vi "ProcAndStates.vi"(0 "spreadsheet string":string) -> (1 "PROCESSES":string[](array[string]), 2 "STATES":string[][](array[string]))   [LabVIEW 2009]
panel:
  out "size(s)":i32[](array[numeric])
  out "Array":string[](array[string])
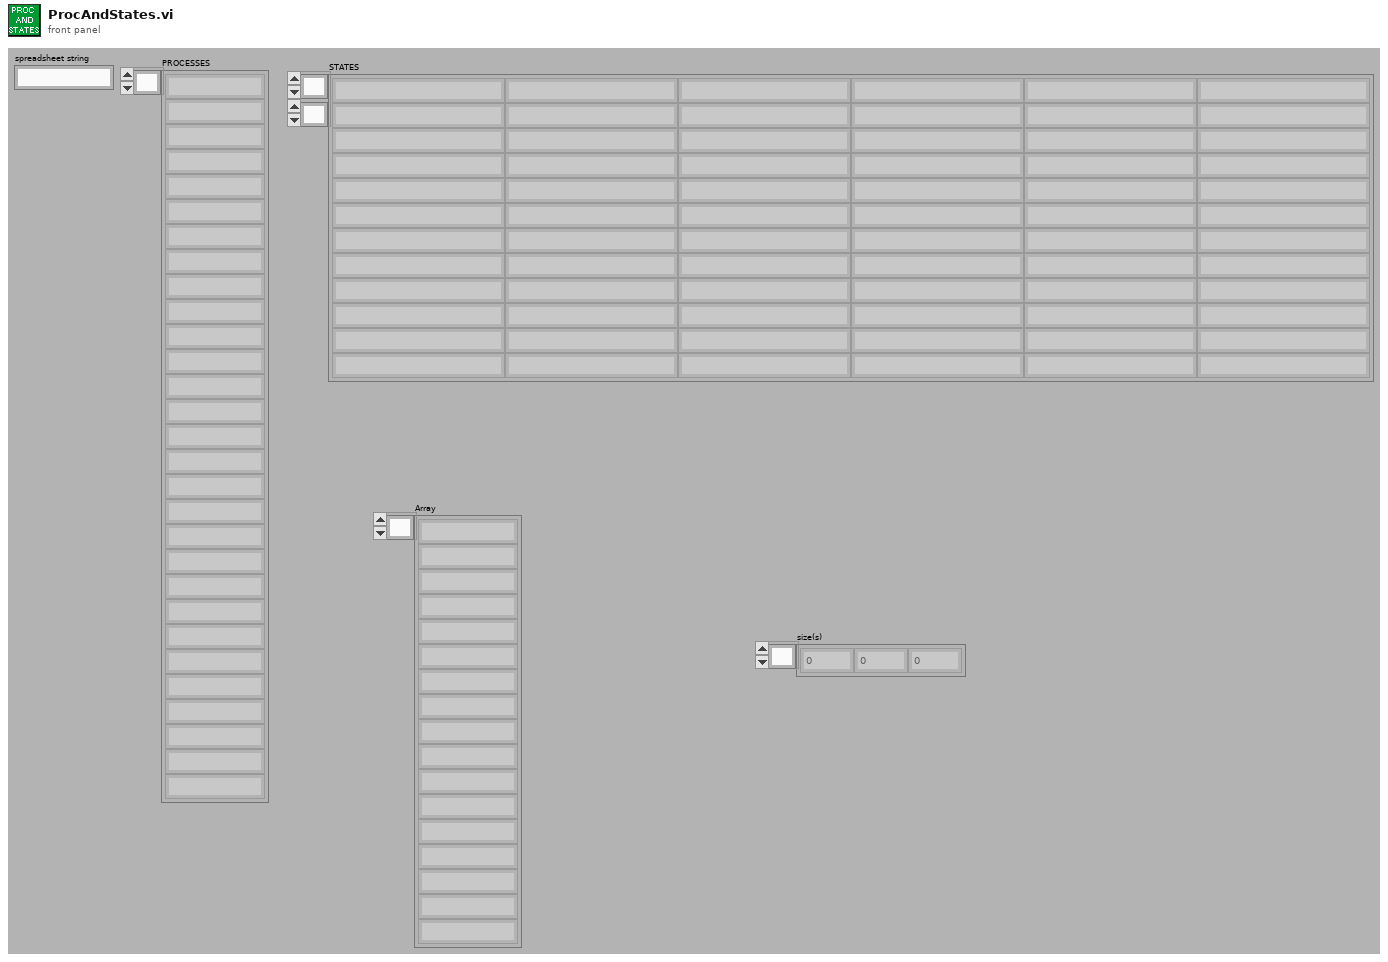
[diagram p1: front panel]
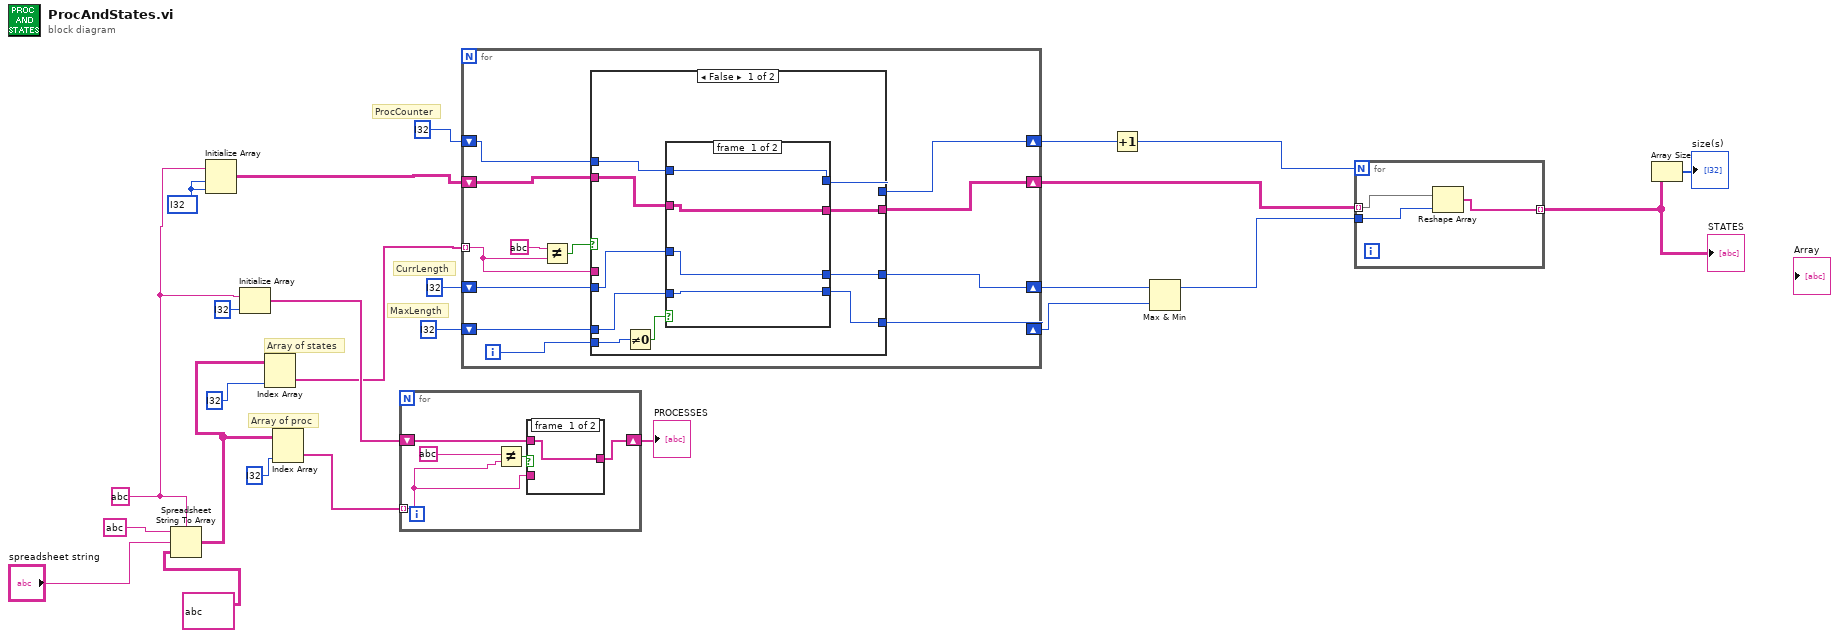
[diagram p0: block diagram]
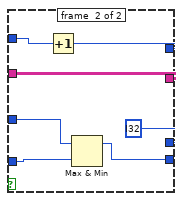
[diagram p2: hidden frame]
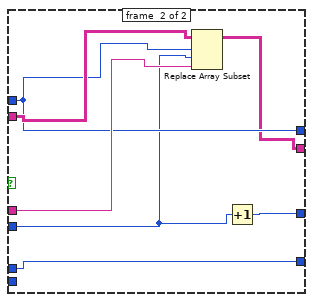
[diagram p3: hidden frame]
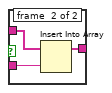
[diagram p4: hidden frame]
diagram:
  w9 = i32 ? ("dimension size")
  w10 = string ? ("delimiter (Tab)")
  # "CurrLength"
  # "MaxLength"
  # "ProcCounter"
  # "Array of proc"
  # "Array of states"
  n1 = Spreadsheet String To Array(delimiter (Tab)=w10, format string=string ?, spreadsheet string="spreadsheet string", array type (2D Dbl)=string[][] ?) -> (array=w24:string[][])
  n2 = Initialize Array(w10, w9, w9) -> (w14:string[][])
  n3 = Initialize Array(w10, i32 ? ("dimension size")) -> (w20:string[])
  n4 = Index Array(array=w24, index (col)=i32 ? ("index (row)")) -> (element=w11:string[])  [unwired: 1 in]
  n5 = Index Array(array=w24, index (col)=i32 ? ("index (row)")) -> (element=w18:string[])  [unwired: 1 in]
  n6 = for {
    tunnel: w18 -> [w29] mode=indexing
    shift-right: [w27] -> w19
    shift-left: w20 -> [w28]
    n7 = Not Equal?(x=string ?, y=w29) -> (x != y?=w30:bool)
    n8 = case shown="True" w30 {
      tunnel: w29 -> [_ w33]
      tunnel: w28 -> [w31 w34]
      tunnel: [w31 w32] -> w27
      frame #0 {
      }
      frame #1 {
        n9 = Insert Into Array(array=w34, new element=w33) -> (w32:string[])  [unwired: 1 in]
      }
    }
  }
  "PROCESSES" <- w19
  n10 = for {
    tunnel: w11 -> [w44] mode=indexing
    shift-right: [w40] -> w6
    shift-left: w14 -> [w45]
    shift-right: [w42] -> w5
    shift-left: i32 ? ("dimension size") -> [w43]
    shift-right: [w39] -> w2
    shift-left: i32 ? ("dimension size") -> [w41]
    shift-right: [w35] -> w3
    shift-left: i32 ? ("dimension size") -> [w36]
    i -> [w37]
    n11 = Not Equal?(x=string ?, y=w44) -> (x != y?=w46:bool)
    n12 = case shown="False" w46 {
      tunnel: [w55 w69] -> w40
      tunnel: w45 -> [w56 w73]
      tunnel: w44 -> [_ w72]
      tunnel: w43 -> [w54 w71]
      tunnel: [w47 w71] -> w42
      tunnel: w41 -> [w53 w74]
      tunnel: [w52 w74] -> w39
      tunnel: w37 -> [w51 _]
      tunnel: w36 -> [w49 w68]
      tunnel: [w48 w70] -> w35
      frame #0 {
        n13 = Not Equal To 0?(x=w51) -> (x != 0?=w50:bool)
        n14 = case shown="True" w50 {
          tunnel: w56 -> [w60 w63]
          tunnel: [w60 w63] -> w55
          tunnel: w54 -> [w58 w67]
          tunnel: [w58 w62] -> w47
          tunnel: w53 -> [w59 w66]
          tunnel: [w59 w61] -> w52
          tunnel: w49 -> [w57 w65]
          tunnel: [w57 i32 ?] -> w48
          frame #0 {
          }
          frame #1 {
            n15 = Increment(x=w67) -> (x+1=w62:i32)
            n16 = Max & Min(x=w65, y=w66) -> (max(x,y)=w61:i32)  [unwired: 1 out]
          }
        }
      }
      frame #1 {
        n17 = Replace Array Subset(array=w73, new element=w72, index (row)=w71, index (col)=w68) -> (w69:string[][])
        n18 = Increment(x=w68) -> (x+1=w70:i32)
      }
    }
  }
  n19 = Increment(x=w5) -> (x+1=w4:i32)
  n20 = Max & Min(x=w3, y=w2) -> (max(x,y)=w1:i32)  [unwired: 1 out]
  n21 = for {
    N: w4 -> [_]
    tunnel: w6 -> [w77] mode=indexing
    tunnel: w1 -> [w76]
    tunnel: [w75] -> w8 mode=indexing
    n22 = Reshape Array(w77, w76) -> (w75:string[])
  }
  "STATES" <- w8
  n23 = Array Size(array=w8) -> (size(s)=→"size(s)":i32[])
